vi "Output_pulse.vi"(8 "error in (no error)":errorcluster, 11 "build_waveform in":refnum<class "build_waveform.lvclass">) -> (0 "error out":errorcluster, 2 "Array":i8[](array[numeric]), 3 "build_waveform out":refnum<class "build_waveform.lvclass">)   [LabVIEW 2019, in "build_waveform.lvclass"]
uses:
  build_waveform.lvclass
  <vilib>/Analysis/NI_AALPro.lvlib
  <vilib>/Analysis/4window.llb/Gaussian Window (DBL).vi
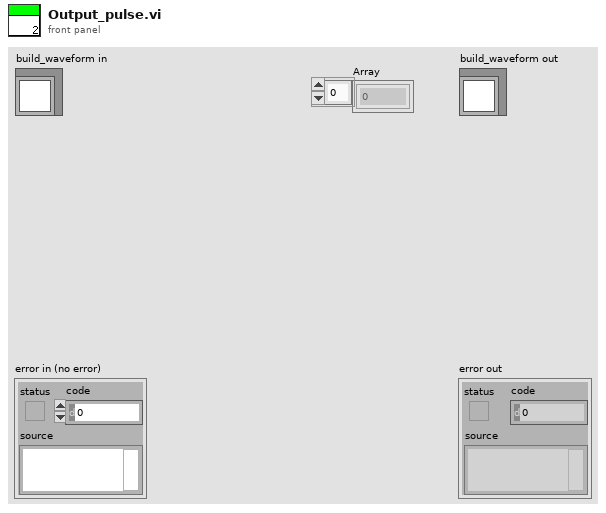
[diagram p1: front panel]
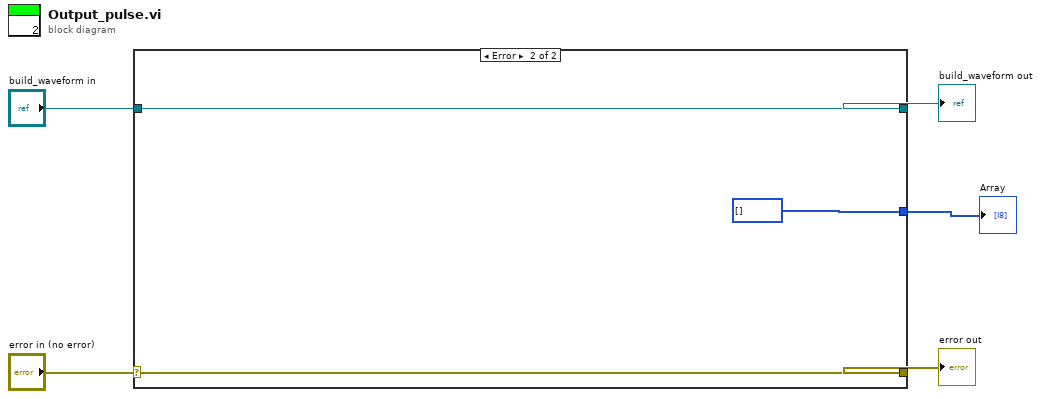
[diagram p0: block diagram]
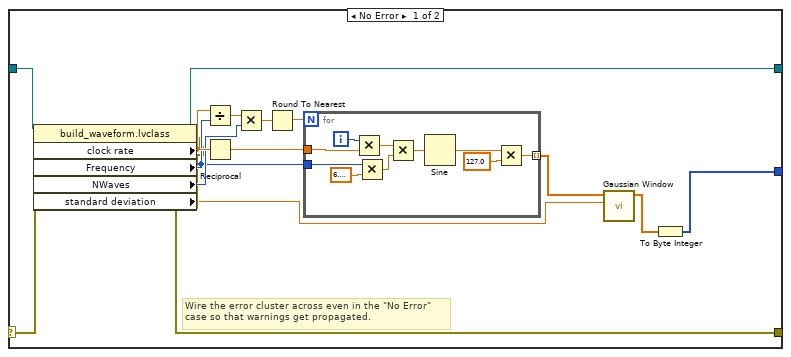
[diagram p2: hidden frame]
diagram:
  n1 = case shown="Error" "error in (no error)" {
    selector: "error in (no error)" -> [w11 w33]
    tunnel: [w10 w33] -> w4
    tunnel: [w12 w32] -> w2
    tunnel: "build_waveform in" -> [w13 w32]
    tunnel: [w6 i8[] []] -> w1
    frame No Error {
      # "Wire the error cluster across even in the \"No Error\"\ncase so that warnings get propagated."
      n2 = property class="build_waveform.lvclass"(reference=w13, error in=w11) -> (reference out=w12:refnum<class "build_waveform.lvclass">, error out=w10:errorcluster, "clock rate"=w20:dbl, "Frequency"=w15:i32, "NWaves"=w19:i32, "standard deviation"=w8:dbl)
      n3 = Divide(x=w20, y=w15) -> (x/y=w18:dbl)
      n4 = Reciprocal(x=w20) -> (1/x=w14:dbl)
      n5 = Multiply(x=w18, y=w19) -> (x*y=w17:dbl)
      n6 = Round To Nearest(number=w17) -> (nearest integer value=w16:dbl)
      n7 = for {
        N: w16 -> [_]
        tunnel: [w24] -> w9 mode=indexing
        tunnel: w15 -> [w21]
        tunnel: w14 -> [w22]
        i -> [w23]
        n8 = Multiply(x=w23, y=w22) -> (x*y=w26:dbl)
        n9 = Multiply(x=w21, y=6.283185307179586) -> (x*y=w27:dbl)
        n10 = Multiply(x=w26, y=w27) -> (x*y=w29:dbl)
        n11 = Sine(x=w29) -> (sin(x)=w25:dbl)
        n12 = Multiply(x=w25, y=127.0) -> (x*y=w24:dbl)
      }
      n13 = call-poly <vilib>:"Gaussian Window.vi"("standard deviation"=w8, "X"=w9) -> ("Windowed X"=w7:dbl[])  [unwired: 8 in, 1 out]
      n14 = To Byte Integer(number=w7) -> (8bit integer=w6:i8[])
    }
    frame Error {
    }
  }
  "error out" <- w4
  "build_waveform out" <- w2
  "Array" <- w1
